vi "Side Ultra Align.vi"() -> (0 "Speed":dbl)   [LabVIEW 2014]
uses:
  TypeDefs/SRE Enum.ctl
panel:
  in  "PD Gains":cluster{"P":dbl, "D":dbl}={"P"=0.02, "D"=0.0}
  in  "Set":dbl=48.0
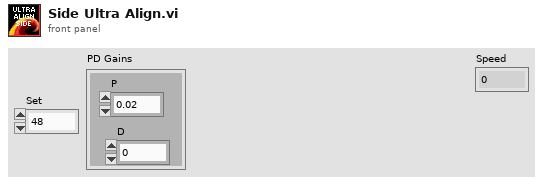
[diagram p1: front panel]
types:
  T1 = typedef "SRE Enum.ctl" = enum16{"Start", "Run", "End"}
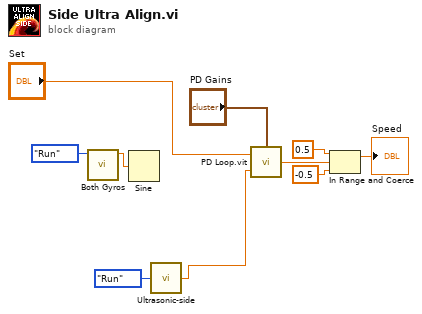
[diagram p0: block diagram]
diagram:
  n1 = call "Both Gyros.vi"("Enum"=SRE_Enum."Run") -> ("Angle"=w2:dbl)  [unwired: 10 in]
  n2 = Sine(x=w2) -> ()  [unwired: 1 out]
  n3 = call "Ultrasonic-side.vi"("Enum"=SRE_Enum."Run") -> ("Distance"=w4:dbl)
  n4 = call "PD Loop.vit"("PD Gains"="PD Gains", "Current"=w4, "Set"="Set") -> ("Out Power"=w7:dbl)
  n5 = In Range and Coerce(upper limit=0.5, x=w7, lower limit=-0.5) -> (coerced(x)=→"Speed":dbl)  [unwired: 1 out]
